vi "_PC_Pub ctrlInterfaceComponent.vi"(7 "This VI":refnum<vi>, 8 "error in (no error)":errorcluster, 11 "Disabled":T1(ring)) -> (0 "error out":errorcluster)   [LabVIEW 2018]
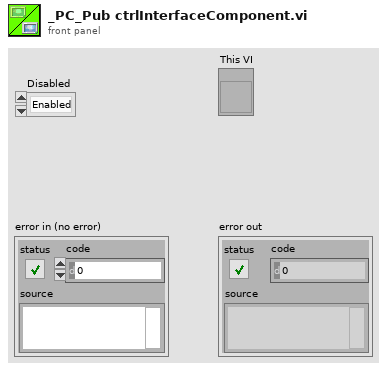
[diagram p1: front panel]
types:
  T1 = enum8{"Enabled", "Disabled", "Disabled and Grayed Out"}
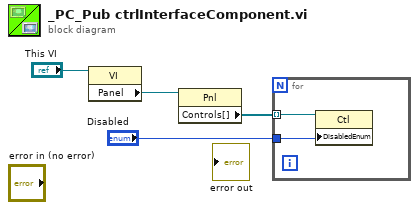
[diagram p0: block diagram]
diagram:
  n1 = property class="VI"(reference="This VI") -> ("Panel"=w3:refnum<vi>)  [unwired: 1 in, 2 out]
  n2 = property class="Pnl"(reference=w3) -> ("Controls[]"=w2:refnum<vi>[])  [unwired: 1 in, 2 out]
  n3 = for {
    tunnel: w2 -> [w6] mode=indexing
    tunnel: "Disabled" -> [w5]
    n4 = property class="Ctl"(reference=w6, "DisabledEnum"=w5) -> ()  [unwired: 1 in, 2 out]
  }
